vi "WIOcompiler.vi"(8 "ino file":path, 10 "hex folder":path, 11 "Java":path) -> (0 "standard error":string, 3 "standard output":string)   [LabVIEW 2020]
uses:
  <vilib>/Utility/sysdir.llb/System Directory Type.ctl
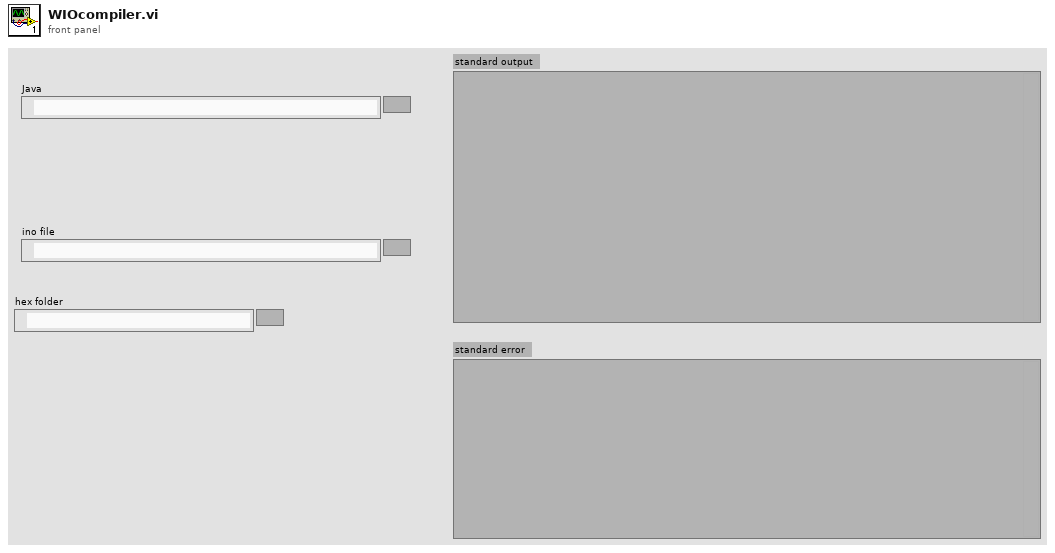
[diagram p1: front panel]
types:
  T1 = typedef "System Directory Type.ctl" = i32
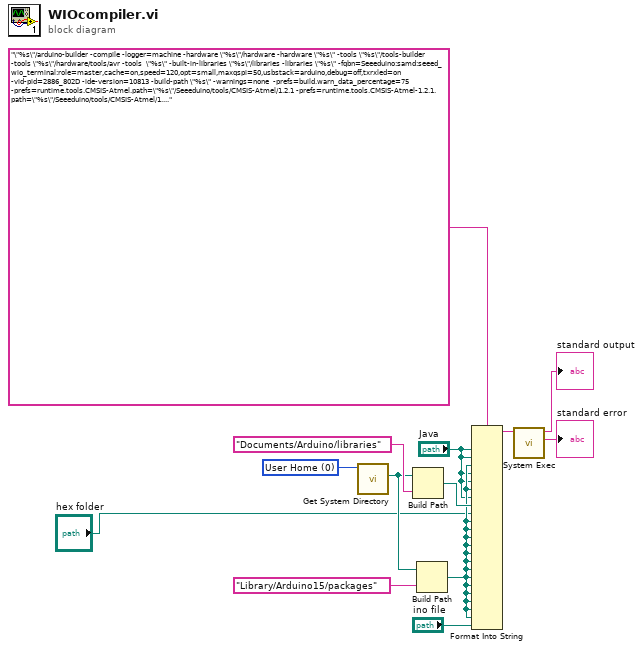
[diagram p0: block diagram]
diagram:
  w10 = T1 0 items=["User Home"=0, "User Desktop"=1, "User Documents"=2, "User Application Data"=3, "User Preferences"=4, "User Temporary"=5, "Public Documents"=6, "Public Application Data"=7, "Public Preferences"=8, "Public Cache"=13, "System Core Libraries"=9, "System Installed Libraries"=10, "Application Files"=11, "Boot Volume Root"=12] ("system directory type")
  n1 = call <vilib>:"Get System Directory.vi"("system directory type"=w10) -> ("system directory"=w6:path)  [unwired: 10 in]
  n2 = Build Path(base path=w6, name or relative path="Documents/Arduino/libraries") -> (appended path=w8:path)
  n3 = Build Path(base path=w6, name or relative path="Library/Arduino15/packages") -> (appended path=w5:path)
  n4 = Format Into String(format string="\"%s\"/arduino-builder -compile -logger=machine -hardware \"%s\"/hardware -hardware \"%s\" -tools \"%s\"/tools-builder -tools \"%s\"/hardware/tools/avr -tools  \"%s\" -built-in-libraries \"%s\"/libraries -libraries \"%s\" -fqbn=Seeeduino:samd:seeed_wio_terminal:role=master,cache=on,speed=120,opt=small,maxqspi=50,usbstack=arduino,debug=off,txrxled=on -vid-pid=2886_802D -ide-version=10813 -build-path \"%s\" -warnings=none  -prefs=build.warn_data_percentage=75 -prefs=runtime.tools.CMSIS-Atmel.path=\"%s\"/Seeeduino/tools/CMSIS-Atmel/1.2.1 -prefs=runtime.tools.CMSIS-Atmel-1.2.1.path=\"%s\"/Seeeduino/tools/CMSIS-Atmel/1.2.1 -prefs=runtime.tools.arduinoOTA.path=\"%s\"/Seeeduino/tools/arduinoOTA/1.2.1 -prefs=runtime.tools.arduinoOTA-1.2.1.path=\"%s\"/Seeeduino/tools/arduinoOTA/1.2.1 -prefs=runtime.tools.bossac.path=\"%s\"/Seeeduino/tools/bossac/1.8.0-48-gb176eee -prefs=runtime.tools.bossac-1.7.0-arduino3.path=\"%s\"/Seeeduino/tools/bossac/1.7.0-arduino3 -prefs=runtime.tools.arm-none-eabi-gcc.path=\"%s\"/Seeeduino/tools/arm-none-eabi-gcc/7-2017q4 -prefs=runtime.tools.arm-none-eabi-gcc-7-2017q4.path=\"%s\"/Seeeduino/tools/arm-none-eabi-gcc/7-2017q4 -prefs=runtime.tools.bossac-1.8.0-48-gb176eee.path=\"%s\"/Seeeduino/tools/bossac/1.8.0-48-gb176eee -prefs=runtime.tools.openocd.path=\"%s\"/arduino/tools/openocd/0.10.0-arduino7 -prefs=runtime.tools.openocd-0.10.0-arduino7.path=\"%s\"/arduino/tools/openocd/0.10.0-arduino7 -prefs=runtime.tools.CMSIS.path=\"%s\"/Seeeduino/tools/CMSIS/5.4.0 -prefs=runtime.tools.CMSIS-5.4.0.path=\"%s\"/Seeeduino/tools/CMSIS/5.4.0 -verbose \"%s\"\n" ("command line"), "Java", "Java", w5, "Java", "Java", w5, "Java", w8, "hex folder", w5, w5, w5, w5, w5, w5, w5, w5, w5, w5, w5, w5, w5, "ino file") -> (resulting string=w4:string)  [unwired: 2 in, 1 out]
  n5 = call <vilib>:"System Exec.vi"("command line"=w4) -> ("standard error"=→"standard error":string, "standard output"=→"standard output":string)  [unwired: 7 in, 2 out]
